vi "ViPER_RenameComponent.vi"(8 "error in (no error)":errorcluster, 9 "Target Path":path, 10 "Component Name":string, 11 "ComponentTemplate":path=path "C:/Program Files (x86)/National Instruments/LabVIEW 2017/ProjectTemplates/Source/Core/ViPER/Components_Src/Component_Template/Component_Template.lvproj") -> (0 "error out":errorcluster)   [LabVIEW 2022 SP3]
uses:
  <vilib>/Utility/lvfile.llb/LVFileType.ctl
  <userlib>/_OpenG.lib/file/file.llb/File Exists - Scalar__ogtk.vi
  <userlib>/_OpenG.lib/file/file.llb/Compare Two Paths - Scalar__ogtk.vi
  <vilib>/Utility/EditLVLibs/Edit LVLibs.lvlib
  <vilib>/Utility/lvfile.llb/NI_FileType.lvlib
panel:
  out "Linker:Read Info From File":T2(array[cluster])
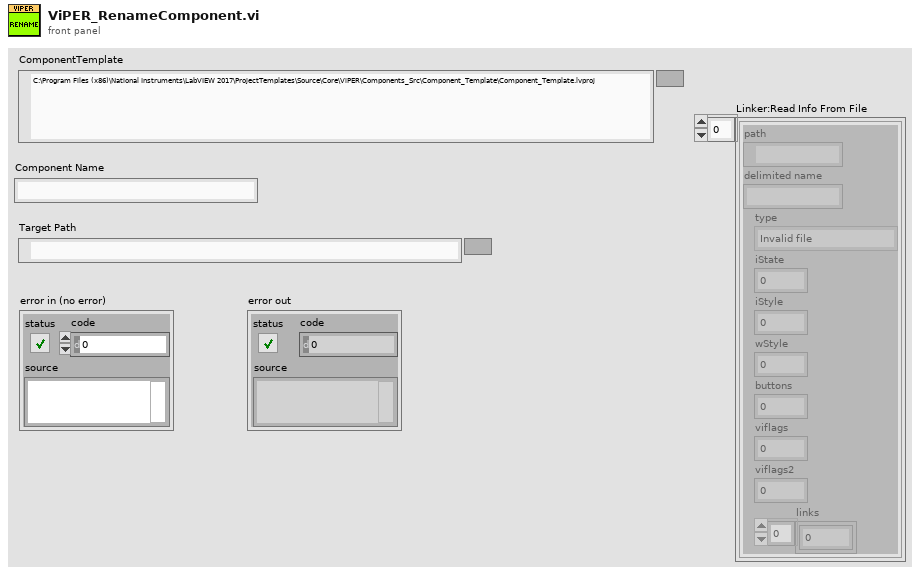
[diagram p1: front panel]
types:
  T1 = typedef "NI_FileType.lvlib/LVFileType.ctl" = enum32{"Invalid file", "Unknown type", "Instrument", "Control", "Polymorphic VI", "Project", "Library", "LVClass", "XControl", "XNode", "Shared library", ".NET assembly", "ActiveX interface", "CIN", "Run-time menu", "Palette menu", "Help file", "LLB", "XNode Edit Dependency", "Class Private Data Control", "Statechart", "MathScript .m file", "Ladder Diagram", "LVLibp", "XNode Build Dependency"}
  T2 = cluster{"path":path, "delimited name":string, "type":T1, "iState":u32, "iStyle":u16, "wStyle":u16, "buttons":u16, "viflags":u32, "viflags2":u32, "links":u32[]}[]
  T3 = cluster{"TempDir":path, "TemplateName":string, "Project":refnum<vi>, "App":refnum<vi>, "SavedProj":path, "TempProj":path, "FinalProj":path, "Linker":cluster{"path":path, "delimited name":string, "type":T1, "iState":u32, "iStyle":u16, "wStyle":u16, "buttons":u16, "viflags":u32, "viflags2":u32, "links":u32[]}[]}
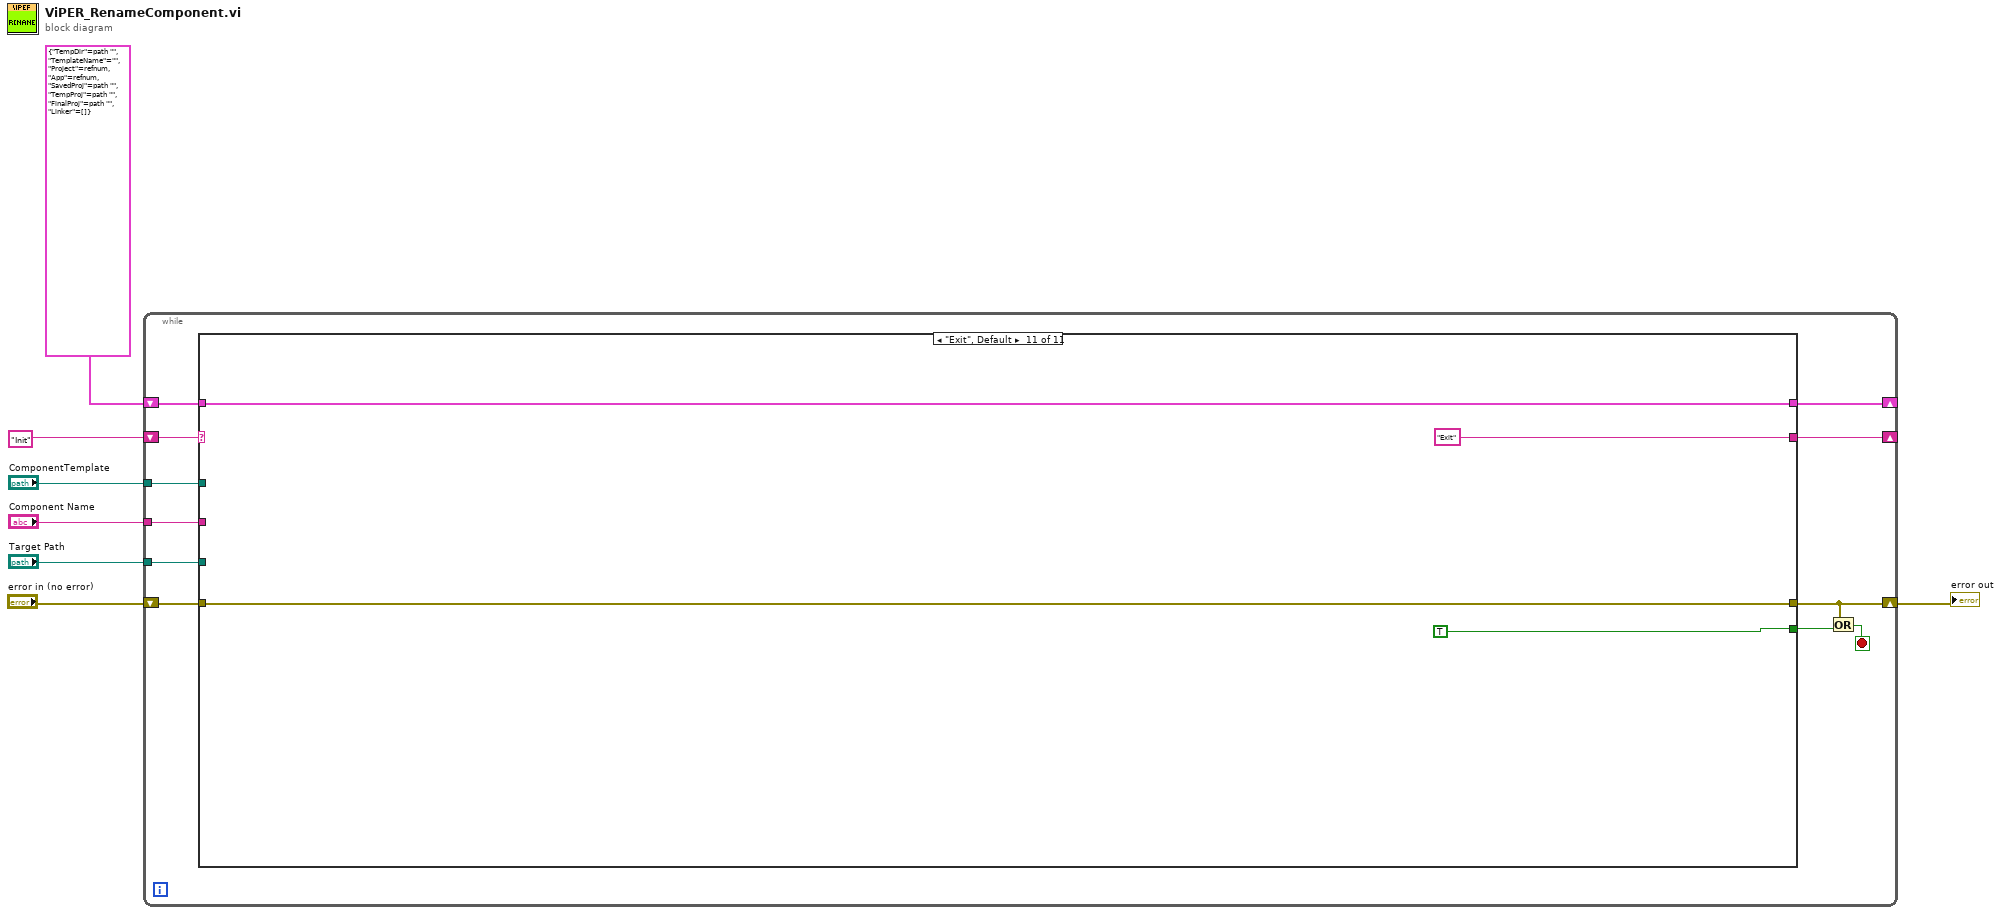
[diagram p0: block diagram]
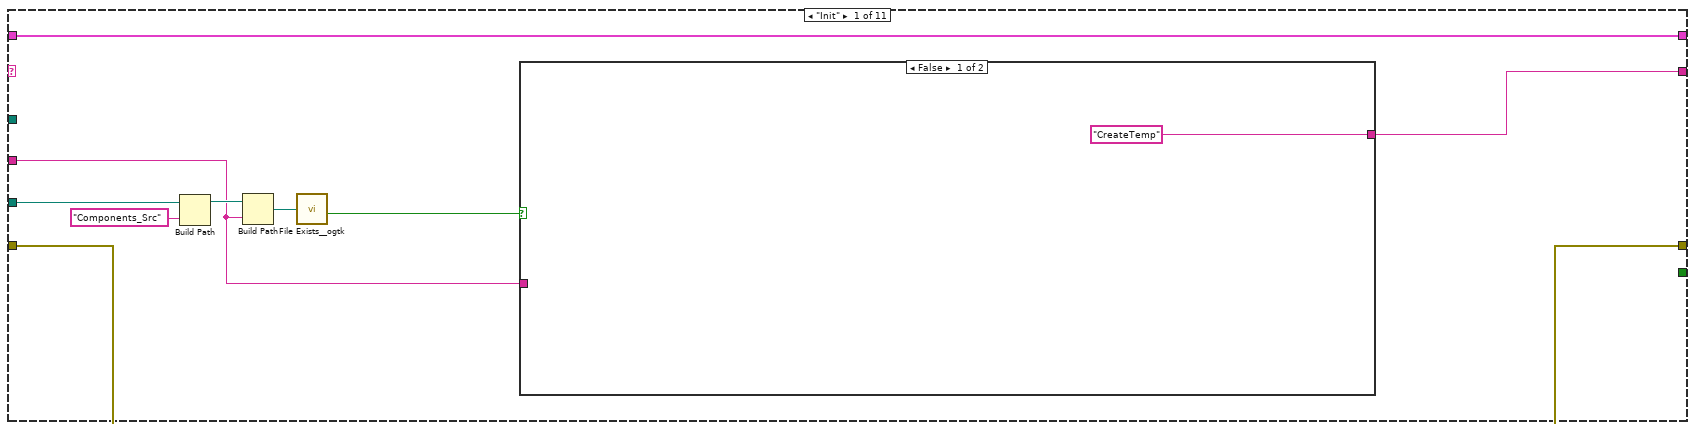
[diagram p2: hidden frame]
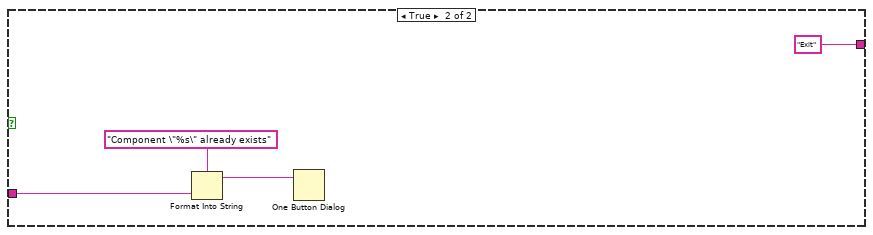
[diagram p3: hidden frame]
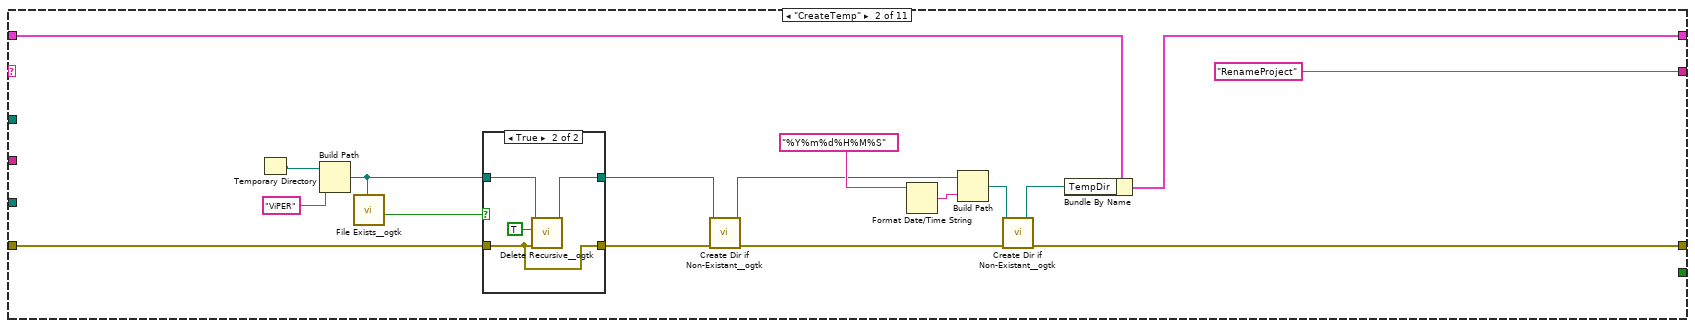
[diagram p4: hidden frame]
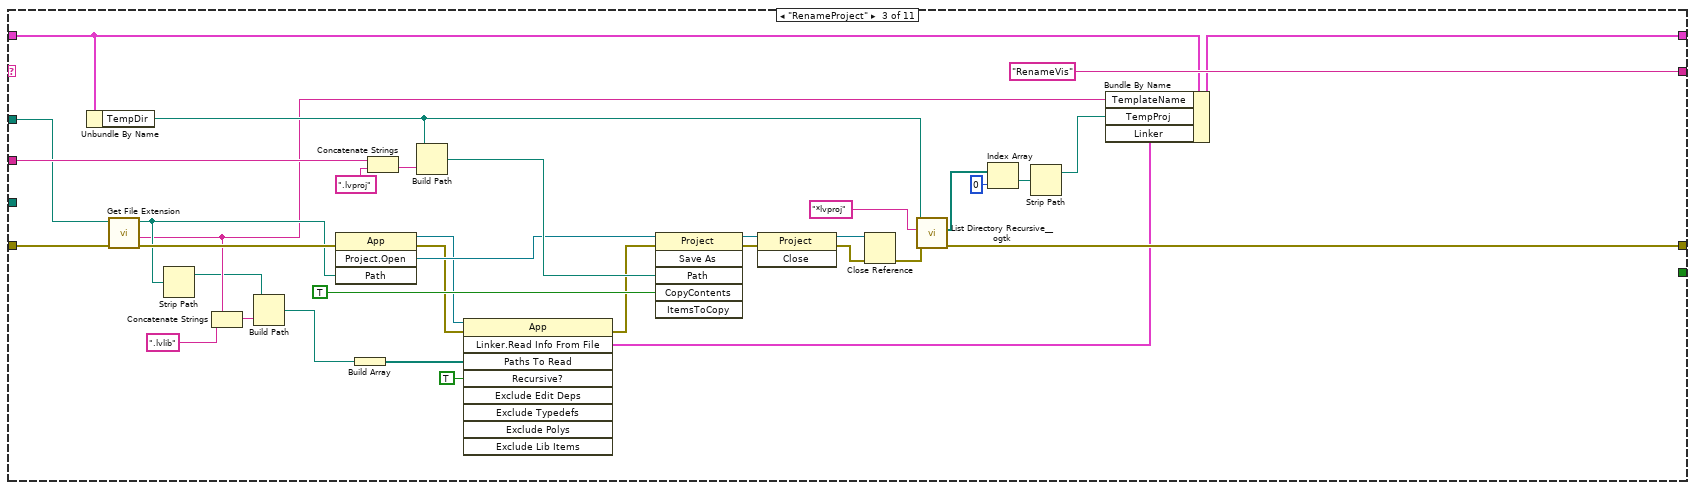
[diagram p6: hidden frame]
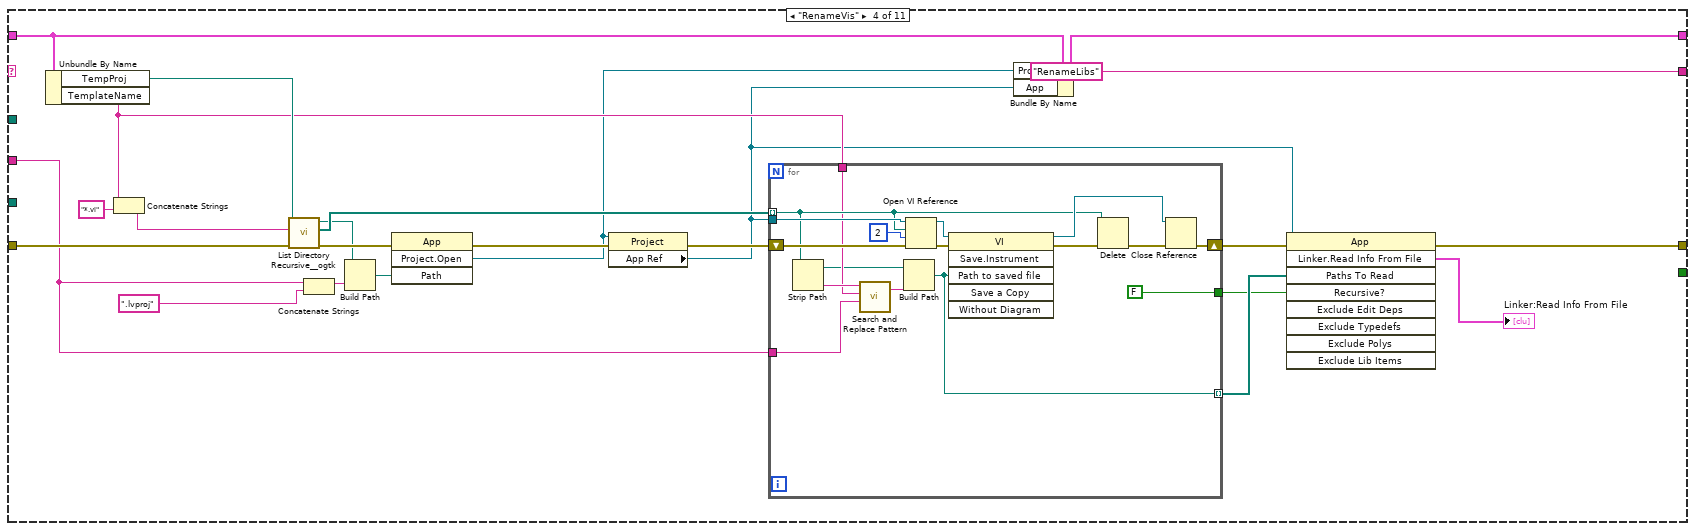
[diagram p7: hidden frame]
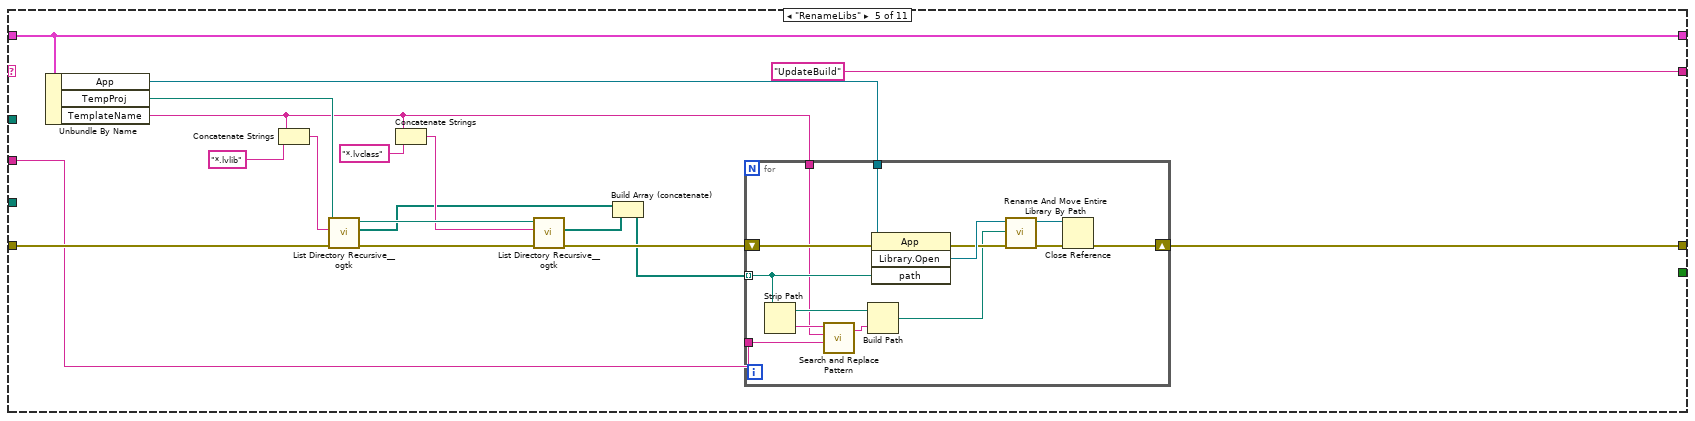
[diagram p8: hidden frame]
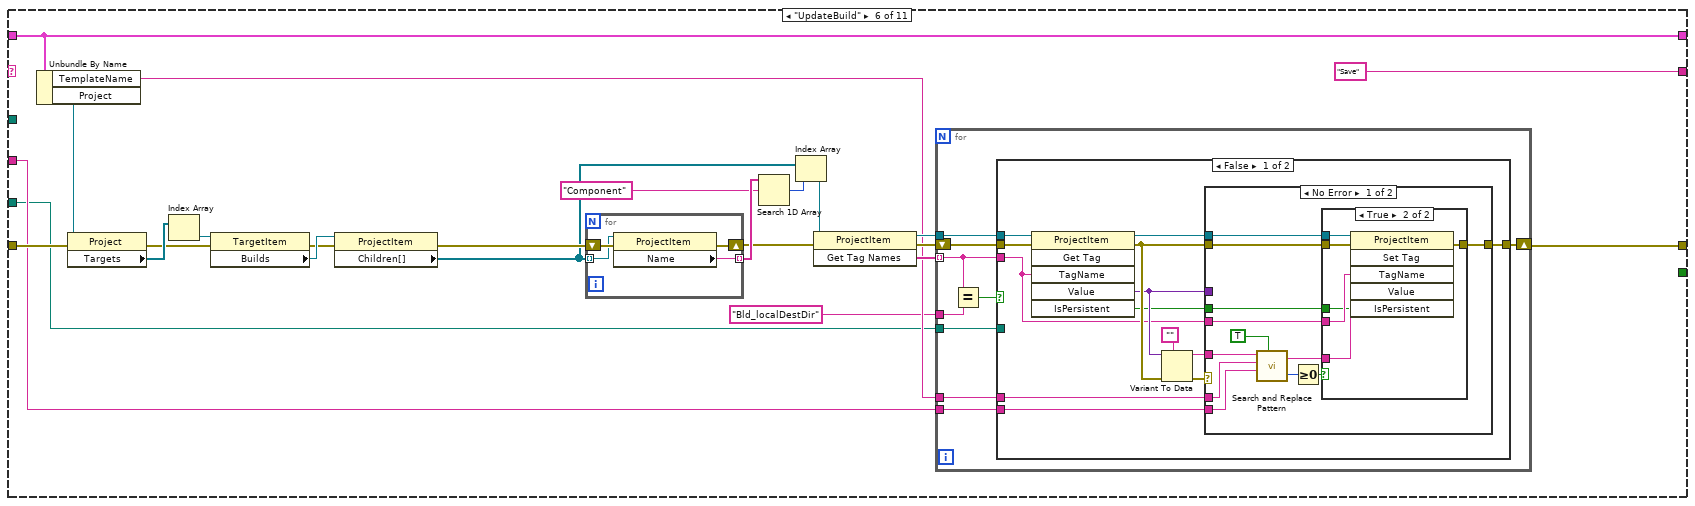
[diagram p9: hidden frame]
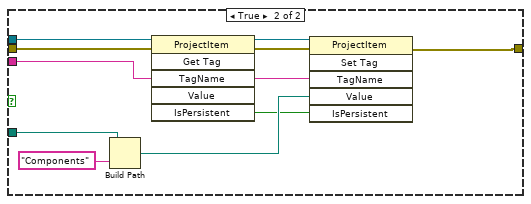
[diagram p12: hidden frame]
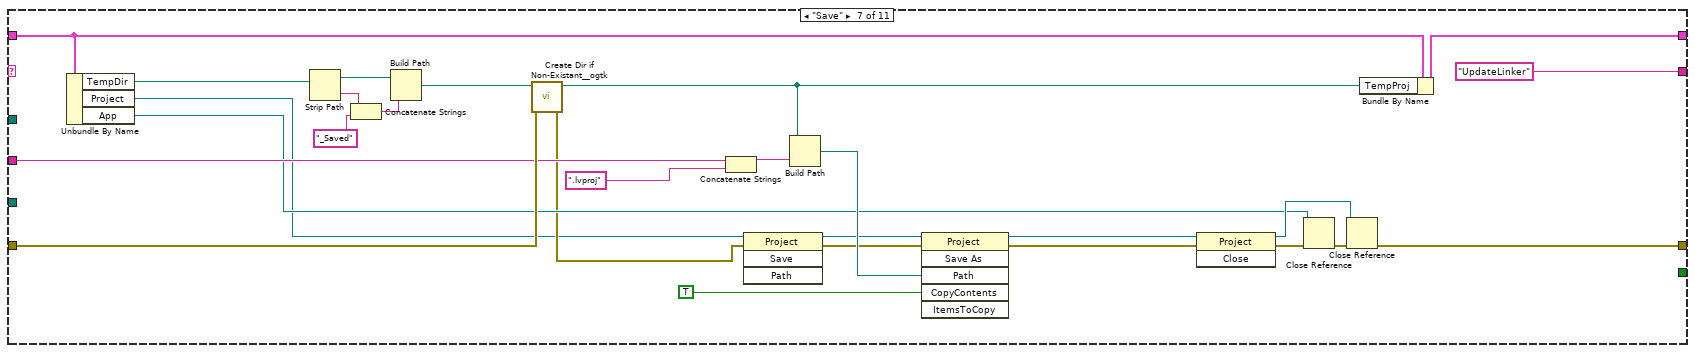
[diagram p13: hidden frame]
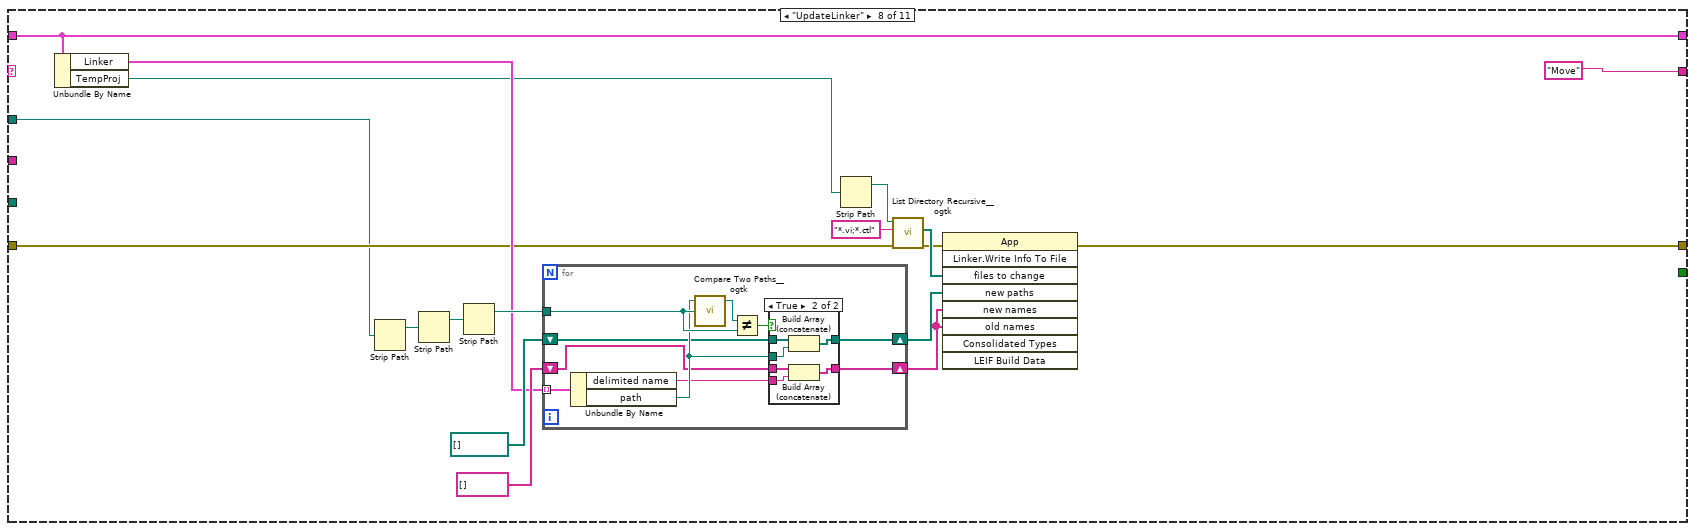
[diagram p14: hidden frame]
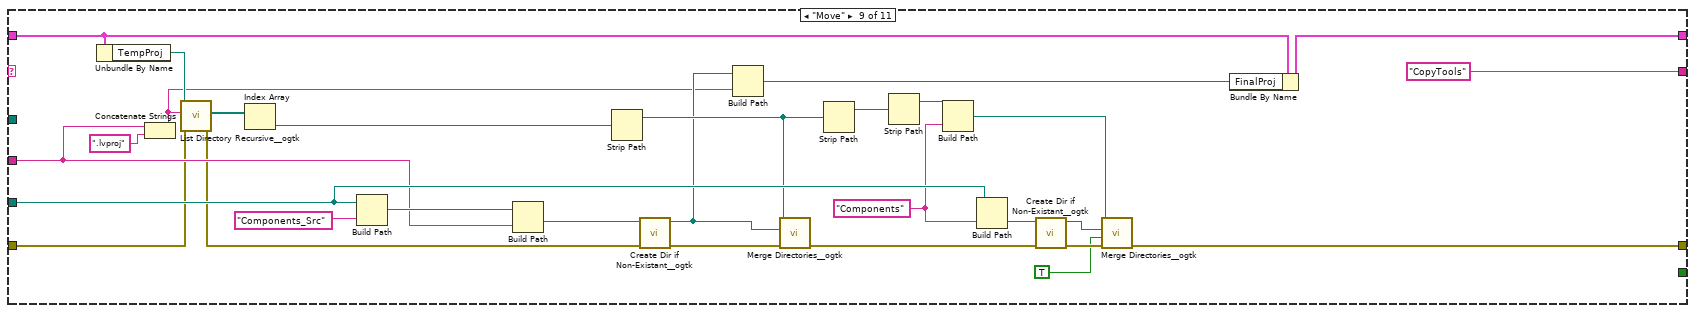
[diagram p16: hidden frame]
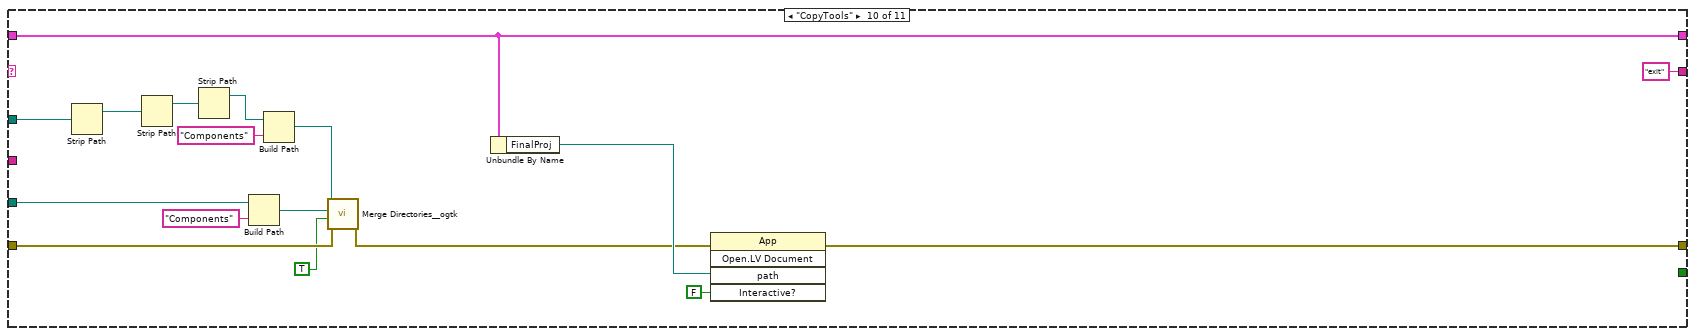
[diagram p17: hidden frame]
diagram:
  n1 = while {
    shift-right: [w15] -> _
    shift-left: T3 {"TempDir"=path "", "TemplateName"="", "Project"=refnum, "App"=refnum, "SavedProj"=path "", "TempProj"=path "", "FinalProj"=path "", "Linker"=[]} -> [w13]
    shift-right: [w14] -> _
    shift-left: "Init" -> [w18]
    tunnel: "ComponentTemplate" -> [w17]
    tunnel: "Component Name" -> [w12]
    shift-right: [w11] -> w1
    shift-left: "error in (no error)" -> [w16]
    tunnel: "Target Path" -> [w9]
    stop <- w10 stop-if-true
    n2 = case shown="\"Exit\", Default" w18 {
      tunnel: w17 -> [_ _ w69 _ _ _ _ w274 _ w353 _]
      tunnel: w16 -> [w20 w45 w71 w113 w149 w179 w264 w276 w319 w344 w356]
      tunnel: [w20 w44 w80 w96 w137 w172 w255 w275 w308 w338 w356] -> w11
      tunnel: [w22 w37 w74 w99 w134 w168 w258 w278 w311 w341 w357] -> w15
      tunnel: [w21 "RenameProject" "RenameVis" "RenameLibs" "UpdateBuild" "Save" "UpdateLinker" "Move" "CopyTools" "exit" "Exit"] -> w14
      tunnel: w13 -> [w22 w39 w75 w100 w134 w168 w260 w278 w312 w341 w357]
      tunnel: w12 -> [w19 _ w86 w102 w135 w170 w263 _ w320 _ _]
      tunnel: w9 -> [w24 _ _ _ _ w165 _ _ w332 w346 _]
      tunnel: [_ _ _ _ _ _ _ _ _ _ TRUE] -> w8
      frame "Init" {
        n3 = Build Path(base path=w24, name or relative path="Components_Src") -> (appended path=w27:path)
        n4 = Build Path(base path=w27, name or relative path=w19) -> (appended path=w26:path)
        n5 = call-poly <userlib>:"File Exists__ogtk.vi"("file path"=w26) -> ("exists"=w23:bool)  [unwired: 6 in, 1 out]
        n6 = case shown="False" w23 {
          tunnel: ["CreateTemp" "Exit"] -> w21
          tunnel: w19 -> [_ w31]
          frame False {
          }
          frame True {
            n7 = Format Into String(format string="Component \"%s\" already exists", w31) -> (resulting string=w29:string)  [unwired: 2 in, 1 out]
            n8 = One Button Dialog(message=w29) -> ()  [unwired: 1 in, 1 out]
          }
        }
      }
      frame "CreateTemp" {
        n9 = Temporary Directory() -> (w49:path)
        n10 = Build Path(base path=w49, name or relative path="ViPER") -> (appended path=w46:path)
        n11 = call-poly <userlib>:"File Exists__ogtk.vi"("file path"=w46) -> ("exists"=w47:bool)  [unwired: 6 in, 1 out]
        n12 = case shown="True" w47 {
          tunnel: w46 -> [w50 w55]
          tunnel: w45 -> [w51 w52]
          tunnel: [w51 w52] -> w36
          tunnel: [w50 w54] -> w33
          frame False {
          }
          frame True {
            n13 = call <userlib>:"Delete Recursive__ogtk.vi"("error in (no error)"=w52, "Recursive? (FALSE)"=TRUE, "Path"=w55) -> ("dup Path"=w54:path)  [unwired: 7 in, 1 out]
          }
        }
        n14 = call <userlib>:"Create Dir if Non-Existant__ogtk.vi"("error in (no error)"=w36, "Directory Path"=w33) -> ("error out"=w35:errorcluster, "dup Directory Path"=w34:path)  [unwired: 7 in, 1 out]
        n15 = Format Date/Time String(time format string (%c)="%Y%m%d%H%M%S") -> (date/time string=w42:string)  [unwired: 2 in]
        n16 = Build Path(base path=w34, name or relative path=w42) -> (appended path=w41:path)
        n17 = call <userlib>:"Create Dir if Non-Existant__ogtk.vi"("error in (no error)"=w35, "Directory Path"=w41) -> ("error out"=w44:errorcluster, "dup Directory Path"=w38:path)  [unwired: 7 in, 1 out]
        n18 = Bundle By Name(cluster=w39, "TempDir"=w38) -> (w37:T3)
      }
      frame "RenameProject" {
        n19 = Unbundle By Name(w75) -> ("TempDir"=w79:path)
        n20 = call <vilib>:"Get File Extension.vi"("error in (no error)"=w71, "file"=w69) -> ("error out"=w70:errorcluster, "filename without extension"=w62:string, "dup file"=w64:path)  [unwired: 5 in, 2 out]
        n21 = Strip Path(path=w64) -> (stripped path=w60:path)  [unwired: 1 out]
        n22 = Concatenate Strings(w62, ".lvlib" ("string")) -> (w61:string)
        n23 = Build Path(base path=w60, name or relative path=w61) -> (appended path=w59:path)
        n24 = invoke class="App" method="Project.Open"(error in=w70, "Path"=w64) -> (reference out=w66:refnum<vi>, error out=w65:errorcluster, "Project:Open"=w67:refnum<vi>)  [unwired: 2 in, 1 out]
        n25 = Build Array(w59) -> (w58:path[])
        n26 = Concatenate Strings(w86, ".lvproj" ("string")) -> (w84:string)
        n27 = Build Path(base path=w79, name or relative path=w84) -> (appended path=w83:path)
        n28 = invoke class="App" method="Linker.Read Info From File"(reference=w66, error in=w65, "Paths To Read"=w58, "Recursive?"=TRUE) -> (error out=w68:errorcluster, "Linker.Read Info From File"=w56:T2)  [unwired: 5 in, 7 out]
        n29 = invoke class="Project" method="Save As"(reference=w67, error in=w68, "Path"=w83, "CopyContents"=TRUE ("Copy contents?")) -> (reference out=w88:refnum<vi>, error out=w90:errorcluster)  [unwired: 2 in, 4 out]
        n30 = invoke class="Project" method="Close"(reference=w88, error in=w90) -> (reference out=w89:refnum<vi>, error out=w91:errorcluster)  [unwired: 1 in, 1 out]
        n31 = Close Reference(reference=w89, error in (no error)=w91) -> (error out=w81:errorcluster)
        n32 = call <userlib>:"List Directory Recursive__ogtk.vi"("error in (no error)"=w81, "pattern"="*lvproj", "Path"=w79) -> ("error out"=w80:errorcluster, "file paths"=w77:path[])  [unwired: 5 in, 2 out]
        n33 = Index Array(array=w77, index=0) -> (element=w73:path)
        n34 = Strip Path(path=w73) -> (stripped path=w72:path)  [unwired: 1 out]
        n35 = Bundle By Name(cluster=w75, "TemplateName"=w62, "TempProj"=w72, "Linker"=w56) -> (w74:T3)
      }
      frame "RenameVis" {
        n36 = Unbundle By Name(w100) -> ("TempProj"=w111:path, "TemplateName"=w103:string)
        n37 = Concatenate Strings(w103, "*.vi" ("string")) -> (w109:string)
        n38 = call <userlib>:"List Directory Recursive__ogtk.vi"("error in (no error)"=w113, "pattern"=w109, "Path"=w111) -> ("error out"=w112:errorcluster, "file paths"=w107:path[], "dup Path"=w105:path)  [unwired: 5 in, 1 out]
        n39 = Concatenate Strings(w102, ".lvproj" ("string")) -> (w106:string)
        n40 = Build Path(base path=w105, name or relative path=w106) -> (appended path=w104:path)
        n41 = invoke class="App" method="Project.Open"(error in=w112, "Path"=w104) -> (error out=w115:errorcluster, "Project:Open"=w98:refnum<vi>)  [unwired: 2 in, 2 out]
        n42 = property class="Project"(reference=w98, error in=w115) -> (error out=w114:errorcluster, "App Ref"=w93:refnum<vi>)  [unwired: 1 out]
        n43 = for {
          tunnel: w107 -> [w125] mode=indexing
          tunnel: w93 -> [w127]
          shift-right: [w128] -> w97
          shift-left: w114 -> [w126]
          tunnel: w103 -> [w123]
          tunnel: w102 -> [w122]
          tunnel: [w117] -> w95 mode=indexing
          tunnel: [FALSE ("Recursive?")] -> w92
          n44 = Strip Path(path=w125) -> (stripped path=w121:path, name=w124:string)
          n45 = call <vilib>:"Search and Replace Pattern.vi"("string"=w124, "regular expression (\"\")"=w123, "replace string (\"\")"=w122) -> ("result string"=w120:string)  [unwired: 2 in, 1 out]
          n46 = Build Path(base path=w121, name or relative path=w120) -> (appended path=w117:path)
          n47 = Open VI Reference(application reference (local)=w127, vi path=w125, options=2 ("Template VIs as templates"), error in (no error)=w126) -> (vi reference=w119:refnum<vi>, error out=w118:errorcluster)  [unwired: 2 in]
          n48 = invoke class="VI" method="Save.Instrument"(reference=w119, error in=w118, "Path to saved file"=w117) -> (reference out=w130:refnum<vi>, error out=w132:errorcluster)  [unwired: 3 in, 4 out]
          n49 = Delete(path (use dialog)=w125, error in=w132) -> (error out=w131:errorcluster)  [unwired: 3 in, 2 out]
          n50 = Close Reference(reference=w130, error in (no error)=w131) -> (error out=w128:errorcluster)
        }
        n51 = Bundle By Name(cluster=w100, "Project"=w98, "App"=w93) -> (w99:T3)
        n52 = invoke class="App" method="Linker.Read Info From File"(reference=w93, error in=w97, "Paths To Read"=w95, "Recursive?"=w92) -> (error out=w96:errorcluster, "Linker.Read Info From File"=→"Linker:Read Info From File":T2)  [unwired: 5 in, 7 out]
      }
      frame "RenameLibs" {
        n53 = Unbundle By Name(w134) -> ("App"=w150:refnum<vi>, "TempProj"=w148:path, "TemplateName"=w136:string)
        n54 = Concatenate Strings(w136, "*.lvlib" ("string")) -> (w146:string)
        n55 = call <userlib>:"List Directory Recursive__ogtk.vi"("error in (no error)"=w149, "pattern"=w146, "Path"=w148) -> ("error out"=w145:errorcluster, "file paths"=w139:path[], "dup Path"=w142:path)  [unwired: 5 in, 1 out]
        n56 = Concatenate Strings(w136, "*.lvclass" ("string")) -> (w141:string)
        n57 = call <userlib>:"List Directory Recursive__ogtk.vi"("error in (no error)"=w145, "pattern"=w141, "Path"=w142) -> ("error out"=w144:errorcluster, "file paths"=w140:path[])  [unwired: 5 in, 2 out]
        n58 = Build Array (concatenate)(w139, w140) -> (w138:path[])
        n59 = for {
          tunnel: w150 -> [w164]
          shift-right: [w151] -> w137
          shift-left: w144 -> [w163]
          tunnel: w138 -> [w157] mode=indexing
          tunnel: w136 -> [w155]
          tunnel: w135 -> [w154]
          n60 = Strip Path(path=w157) -> (stripped path=w159:path, name=w160:string)
          n61 = call <vilib>:"Search and Replace Pattern.vi"("string"=w160, "regular expression (\"\")"=w155, "replace string (\"\")"=w154) -> ("result string"=w158:string)  [unwired: 2 in, 1 out]
          n62 = Build Path(base path=w159, name or relative path=w158) -> (appended path=w156:path)
          n63 = invoke class="App" method="Library.Open"(reference=w164, error in=w163, "path"=w157) -> (error out=w161:errorcluster, "Open Library"=w162:refnum<vi>)  [unwired: 1 in, 2 out]
          n64 = call <vilib>:"Rename And Move Entire Library By Path.vi"("error in (no error)"=w161, "New library path"=w156, "Library ref in"=w162) -> ("error out"=w152:errorcluster, "Library ref out"=w153:refnum<vi>)  [unwired: 7 in]
          n65 = Close Reference(reference=w153, error in (no error)=w152) -> (error out=w151:errorcluster)
        }
      }
      frame "UpdateBuild" {
        n66 = Unbundle By Name(w168) -> ("TemplateName"=w169:string, "Project"=w178:refnum<vi>)
        n67 = property class="Project"(reference=w178, error in=w179) -> (error out=w186:errorcluster, "Targets"=w188:refnum<vi>[])  [unwired: 1 out]
        n68 = Index Array(array=w188) -> (element=w187:refnum<vi>)  [unwired: 1 in]
        n69 = property class="TargetItem"(reference=w187, error in=w186) -> (error out=w184:errorcluster, "Builds"=w185:refnum<vi>)  [unwired: 1 out]
        n70 = property class="ProjectItem"(reference=w185, error in=w184) -> (error out=w182:errorcluster, "Children[]"=w181:refnum<vi>[])  [unwired: 1 out]
        n71 = for {
          tunnel: w181 -> [w243] mode=indexing
          shift-right: [w242] -> w173
          shift-left: w182 -> [w244]
          tunnel: [w241] -> w183 mode=indexing
          n72 = property class="ProjectItem"(reference=w243, error in=w244) -> (error out=w242:errorcluster, "Name"=w241:string)  [unwired: 1 out]
        }
        n73 = Search 1D Array(1D array=w183, element="Component") -> (index of element=w180:i32)  [unwired: 1 in]
        n74 = Index Array(array=w181, index=w180) -> (element=w174:refnum<vi>)
        n75 = invoke class="ProjectItem" method="Get Tag Names"(reference=w174, error in=w173) -> (reference out=w176:refnum<vi>, error out=w175:errorcluster, "Get Tag Names"=w177:string[])  [unwired: 1 in]
        n76 = for {
          tunnel: w177 -> [w191] mode=indexing
          tunnel: w176 -> [w197]
          tunnel: w169 -> [w194]
          tunnel: w170 -> [w193]
          shift-right: [w195] -> w172
          shift-left: w175 -> [w196]
          tunnel: "Bld_localDestDir" ("element") -> [w192]
          tunnel: w165 -> [w189]
          n77 = Equal?(x=w191, y=w192) -> (x = y?=w190:bool)
          n78 = case shown="False" w190 {
            tunnel: w197 -> [w210 w238]
            tunnel: w196 -> [w208 w237]
            tunnel: [w207 w231] -> w195
            tunnel: w194 -> [w203 _]
            tunnel: w193 -> [w202 _]
            tunnel: w191 -> [w199 w234]
            tunnel: w189 -> [_ w239]
            frame False {
              n79 = invoke class="ProjectItem" method="Get Tag"(reference=w210, error in=w208, "TagName"=w199) -> (reference out=w209:refnum<vi>, error out=w204:errorcluster, "Value"=w200:variant, "IsPersistent"=w198:bool)  [unwired: 3 in, 2 out]
              n80 = Variant To Data(error in=w204, type="", Variant=w200) -> (data=w201:string, error out=w205:errorcluster)
              n81 = case shown="No Error" w205 {
                tunnel: w209 -> [w222 _]
                tunnel: w199 -> [w215 _]
                tunnel: w204 -> [w221 w230]
                tunnel: [w220 w230] -> w207
                tunnel: w203 -> [w219 _]
                tunnel: w202 -> [w218 _]
                tunnel: w201 -> [w216 _]
                tunnel: w200 -> [_ _]
                tunnel: w198 -> [w211 _]
                frame No Error {
                  n82 = call <vilib>:"Search and Replace Pattern.vi"("string"=w216, "regular expression (\"\")"=w219, "replace string (\"\")"=w218, "replace all? (F)"=TRUE) -> ("result string"=w212:string, "offset past match"=w214:i32)  [unwired: 1 in]
                  n83 = Greater Or Equal To 0?(x=w214) -> (x >= 0?=w213:bool)
                  n84 = case shown="True" w213 {
                    tunnel: w222 -> [_ w229]
                    tunnel: w221 -> [w223 w228]
                    tunnel: [w223 w227] -> w220
                    tunnel: w215 -> [_ w226]
                    tunnel: w212 -> [_ w225]
                    tunnel: w211 -> [_ w224]
                    frame False {
                    }
                    frame True {
                      n85 = invoke class="ProjectItem" method="Set Tag"(reference=w229, error in=w228, "TagName"=w226, "Value"=w225, "IsPersistent"=w224) -> (error out=w227:errorcluster)  [unwired: 1 in, 5 out]
                    }
                  }
                }
                frame Error {
                }
              }
            }
            frame True {
              n86 = Build Path(base path=w239, name or relative path="Components") -> (appended path=w233:path)
              n87 = invoke class="ProjectItem" method="Get Tag"(reference=w238, error in=w237, "TagName"=w234) -> (reference out=w236:refnum<vi>, error out=w235:errorcluster, "IsPersistent"=w232:bool)  [unwired: 3 in, 3 out]
              n88 = invoke class="ProjectItem" method="Set Tag"(reference=w236, error in=w235, "TagName"=w234, "Value"=w233, "IsPersistent"=w232) -> (error out=w231:errorcluster)  [unwired: 1 in, 5 out]
            }
          }
        }
      }
      frame "Save" {
        n89 = Unbundle By Name(w260) -> ("TempDir"=w270:path, "Project"=w246:refnum<vi>, "App"=w252:refnum<vi>)
        n90 = Strip Path(path=w270) -> (stripped path=w269:path, name=w268:string)
        n91 = Concatenate Strings(w268, "_Saved" ("string")) -> (w253:string)
        n92 = Build Path(base path=w269, name or relative path=w253) -> (appended path=w265:path)
        n93 = call <userlib>:"Create Dir if Non-Existant__ogtk.vi"("error in (no error)"=w264, "Directory Path"=w265) -> ("error out"=w247:errorcluster, "dup Directory Path"=w259:path)  [unwired: 7 in, 1 out]
        n94 = Concatenate Strings(w263, ".lvproj" ("string")) -> (w262:string)
        n95 = invoke class="Project" method="Save"(reference=w246, error in=w247) -> (reference out=w251:refnum<vi>, error out=w250:errorcluster)  [unwired: 2 in, 2 out]
        n96 = Build Path(base path=w259, name or relative path=w262) -> (appended path=w261:path)
        n97 = invoke class="Project" method="Save As"(reference=w251, error in=w250, "Path"=w261, "CopyContents"=TRUE ("Copy contents?")) -> (reference out=w249:refnum<vi>, error out=w248:errorcluster)  [unwired: 2 in, 4 out]
        n98 = invoke class="Project" method="Close"(reference=w249, error in=w248) -> (reference out=w254:refnum<vi>, error out=w256:errorcluster)  [unwired: 1 in, 1 out]
        n99 = Close Reference(reference=w252, error in (no error)=w256) -> (error out=w257:errorcluster)
        n100 = Close Reference(reference=w254, error in (no error)=w257) -> (error out=w255:errorcluster)
        n101 = Bundle By Name(cluster=w260, "TempProj"=w259) -> (w258:T3)
      }
      frame "UpdateLinker" {
        n102 = Unbundle By Name(w278) -> ("Linker"=w277:T2, "TempProj"=w272:path)
        n103 = Strip Path(path=w274) -> (stripped path=w287:path)  [unwired: 1 out]
        n104 = Strip Path(path=w287) -> (stripped path=w288:path)  [unwired: 1 out]
        n105 = Strip Path(path=w288) -> (stripped path=w283:path)  [unwired: 1 out]
        n106 = for {
          tunnel: w277 -> [w299] mode=indexing
          tunnel: w283 -> [w297]
          shift-right: [w294] -> w279
          shift-left: path[] [] -> [w293]
          shift-right: [w291] -> w280
          shift-left: string[] [] -> [w290]
          n107 = Unbundle By Name(w299) -> ("delimited name"=w292:string, "path"=w295:path)
          n108 = call-poly <userlib>:"Compare Two Paths__ogtk.vi"("path2"=w297, "path1"=w295) -> ("common path"=w298:path)  [unwired: 1 in, 2 out]
          n109 = Not Equal?(x=w298, y=w297) -> (x != y?=w296:bool)
          n110 = case shown="True" w296 {
            tunnel: w295 -> [_ w307]
            tunnel: [w300 w306] -> w294
            tunnel: w293 -> [w300 w305]
            tunnel: w292 -> [_ w304]
            tunnel: [w301 w303] -> w291
            tunnel: w290 -> [w301 w302]
            frame False {
            }
            frame True {
              n111 = Build Array (concatenate)(w305, w307) -> (w306:path[])
              n112 = Build Array (concatenate)(w302, w304) -> (w303:string[])
            }
          }
        }
        n113 = Strip Path(path=w272) -> (stripped path=w284:path)  [unwired: 1 out]
        n114 = call <userlib>:"List Directory Recursive__ogtk.vi"("error in (no error)"=w276, "pattern"="*.vi;*.ctl", "Path"=w284) -> ("error out"=w285:errorcluster, "file paths"=w286:path[])  [unwired: 5 in, 2 out]
        n115 = invoke class="App" method="Linker.Write Info To File"(error in=w285, "files to change"=w286, "new paths"=w279, "new names"=w280, "old names"=w280) -> (error out=w275:errorcluster)  [unwired: 4 in, 8 out]
      }
      frame "Move" {
        w324 = "Components" ("name or relative path")
        n116 = Unbundle By Name(w312) -> ("TempProj"=w322:path)
        n117 = Concatenate Strings(w320, ".lvproj" ("string")) -> (w313:string)
        n118 = call <userlib>:"List Directory Recursive__ogtk.vi"("error in (no error)"=w319, "pattern"=w313, "Path"=w322) -> ("error out"=w318:errorcluster, "file paths"=w317:path[])  [unwired: 5 in, 2 out]
        n119 = Index Array(array=w317) -> (element=w315:path)  [unwired: 1 in]
        n120 = Build Path(base path=w332, name or relative path="Components_Src") -> (appended path=w335:path)
        n121 = Build Path(base path=w335, name or relative path=w320) -> (appended path=w334:path)
        n122 = Strip Path(path=w315) -> (stripped path=w329:path)  [unwired: 1 out]
        n123 = call <userlib>:"Create Dir if Non-Existant__ogtk.vi"("error in (no error)"=w318, "Directory Path"=w334) -> ("error out"=w333:errorcluster, "dup Directory Path"=w314:path)  [unwired: 7 in, 1 out]
        n124 = Build Path(base path=w314, name or relative path=w313) -> (appended path=w309:path)
        n125 = call <userlib>:"Merge Directories__ogtk.vi"("error in (no error)"=w333, "target directory path"=w314, "source directory path"=w329) -> ("error out"=w331:errorcluster)  [unwired: 7 in, 1 out]
        n126 = Strip Path(path=w329) -> (stripped path=w326:path)  [unwired: 1 out]
        n127 = Strip Path(path=w326) -> (stripped path=w325:path)  [unwired: 1 out]
        n128 = Build Path(base path=w325, name or relative path=w324) -> (appended path=w323:path)
        n129 = Build Path(base path=w332, name or relative path=w324) -> (appended path=w330:path)
        n130 = call <userlib>:"Create Dir if Non-Existant__ogtk.vi"("error in (no error)"=w331, "Directory Path"=w330) -> ("error out"=w328:errorcluster, "dup Directory Path"=w327:path)  [unwired: 7 in, 1 out]
        n131 = call <userlib>:"Merge Directories__ogtk.vi"("error in (no error)"=w328, "Overwrite Existing Files? (FALSE)"=TRUE, "target directory path"=w327, "source directory path"=w323) -> ("error out"=w308:errorcluster)  [unwired: 6 in, 1 out]
        n132 = Bundle By Name(cluster=w312, "FinalProj"=w309) -> (w311:T3)
      }
      frame "CopyTools" {
        n133 = Strip Path(path=w353) -> (stripped path=w352:path)  [unwired: 1 out]
        n134 = Strip Path(path=w352) -> (stripped path=w351:path)  [unwired: 1 out]
        n135 = Strip Path(path=w351) -> (stripped path=w350:path)  [unwired: 1 out]
        n136 = Build Path(base path=w346, name or relative path="Components") -> (appended path=w345:path)
        n137 = Build Path(base path=w350, name or relative path="Components") -> (appended path=w348:path)
        n138 = call <userlib>:"Merge Directories__ogtk.vi"("error in (no error)"=w344, "Overwrite Existing Files? (FALSE)"=TRUE, "target directory path"=w345, "source directory path"=w348) -> ("error out"=w339:errorcluster)  [unwired: 6 in, 1 out]
        n139 = Unbundle By Name(w341) -> ("FinalProj"=w340:path)
        n140 = invoke class="App" method="Open.LV Document"(error in=w339, "path"=w340, "Interactive?"=FALSE) -> (error out=w338:errorcluster)  [unwired: 2 in, 4 out]
      }
      frame "Exit", Default {
      }
    }
    n141 = Or(x=w11, y=w8) -> (x .or. y?=w10:bool)
  }
  "error out" <- w1
